vi "VariantSelection.vi"(8 "error in (no error)":errorcluster) -> (0 "error out":errorcluster, 2 "Cancelled":bool)   [LabVIEW 2013]
uses:
  <vilib>/addons/database/NI_Database_API.lvlib
  VariableLIB/Global.vi
  <vilib>/addons/database/Connection.llb/DB Tools Open Connec (String).vi
  Controls/AppleButton.ctl
panel:
  in  "Cancel":T1
  in  "Part":i32(ring) items=["HF DELUXE", "SPLENDOR PRO", "HF DELUXE WITH SIDE STAND", "SPLENDOR PRO WITH SIDE STAND", "CD DELUXE", "AAHC"]
  in  "OK":T1
  in  "Model":i32(ring) items=["AAHC", "DEFAULT MODEL", "HMCL"]
  # "Variant selection"
  # "Select a model"
  # "Select a part"
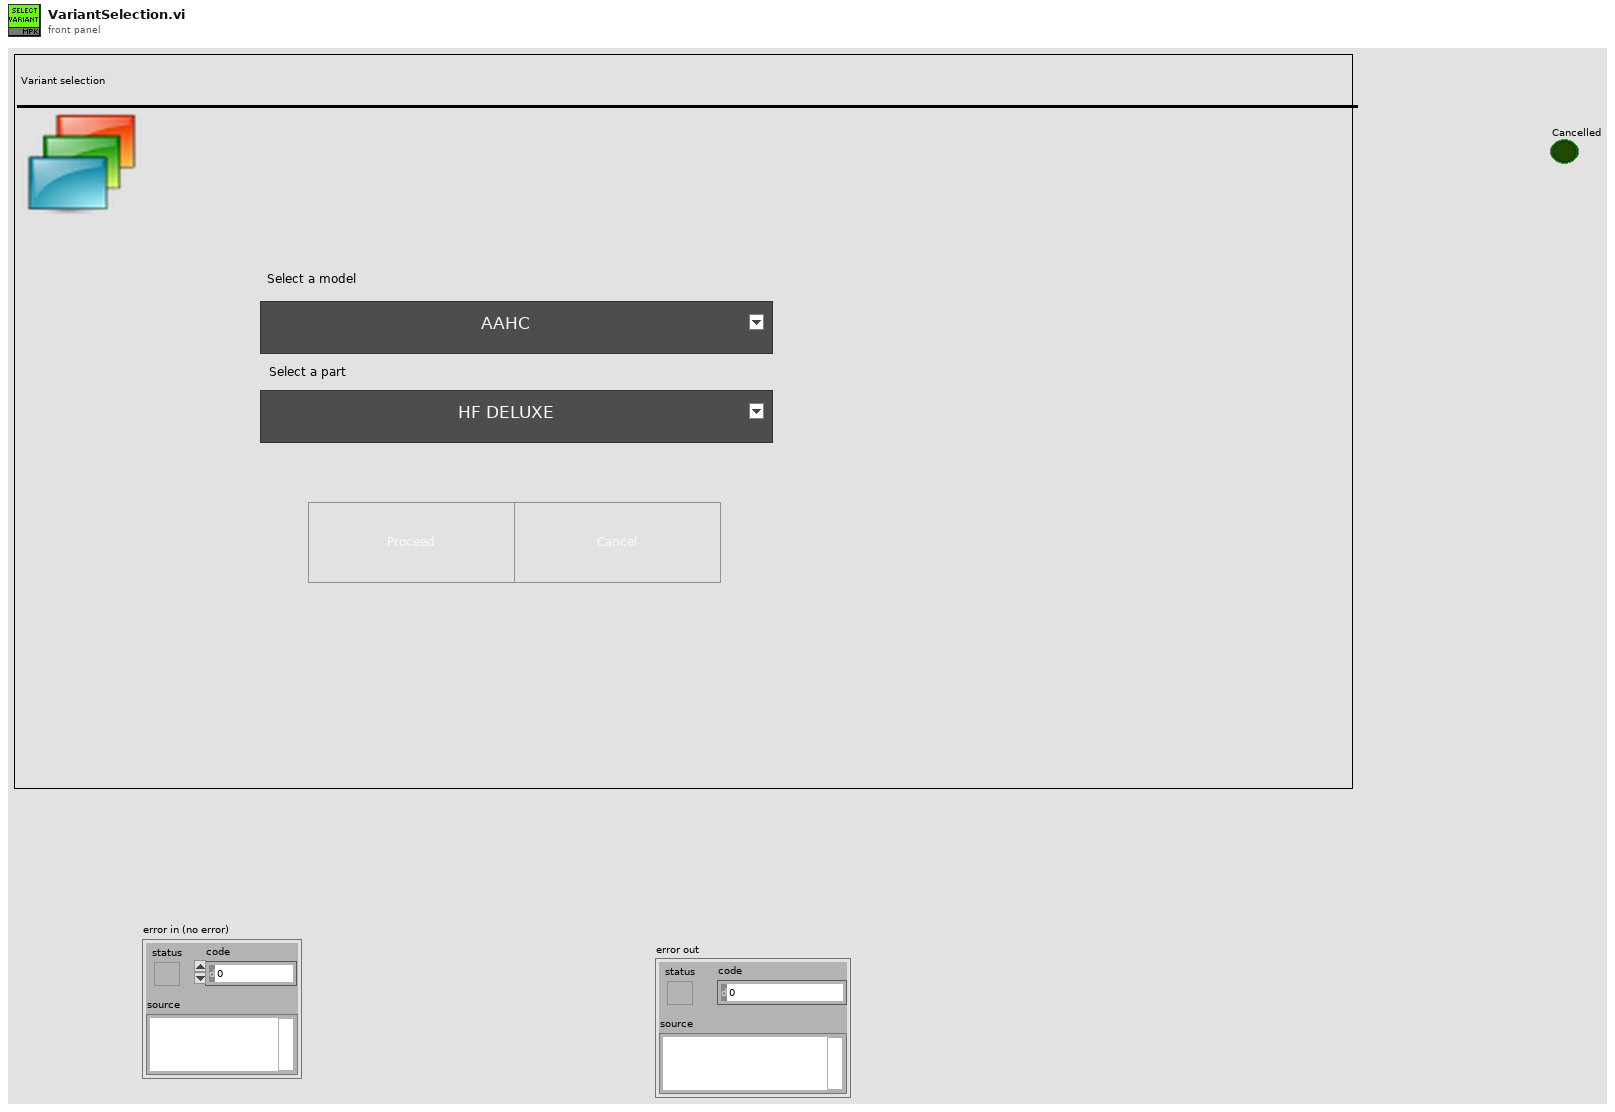
[diagram p1: front panel]
types:
  T1 = typedef "AppleButton.ctl" = bool
  T2 = typedef "NI_Database_API.lvlib/Conn ObjectReference.ctl" = refnum<k1>
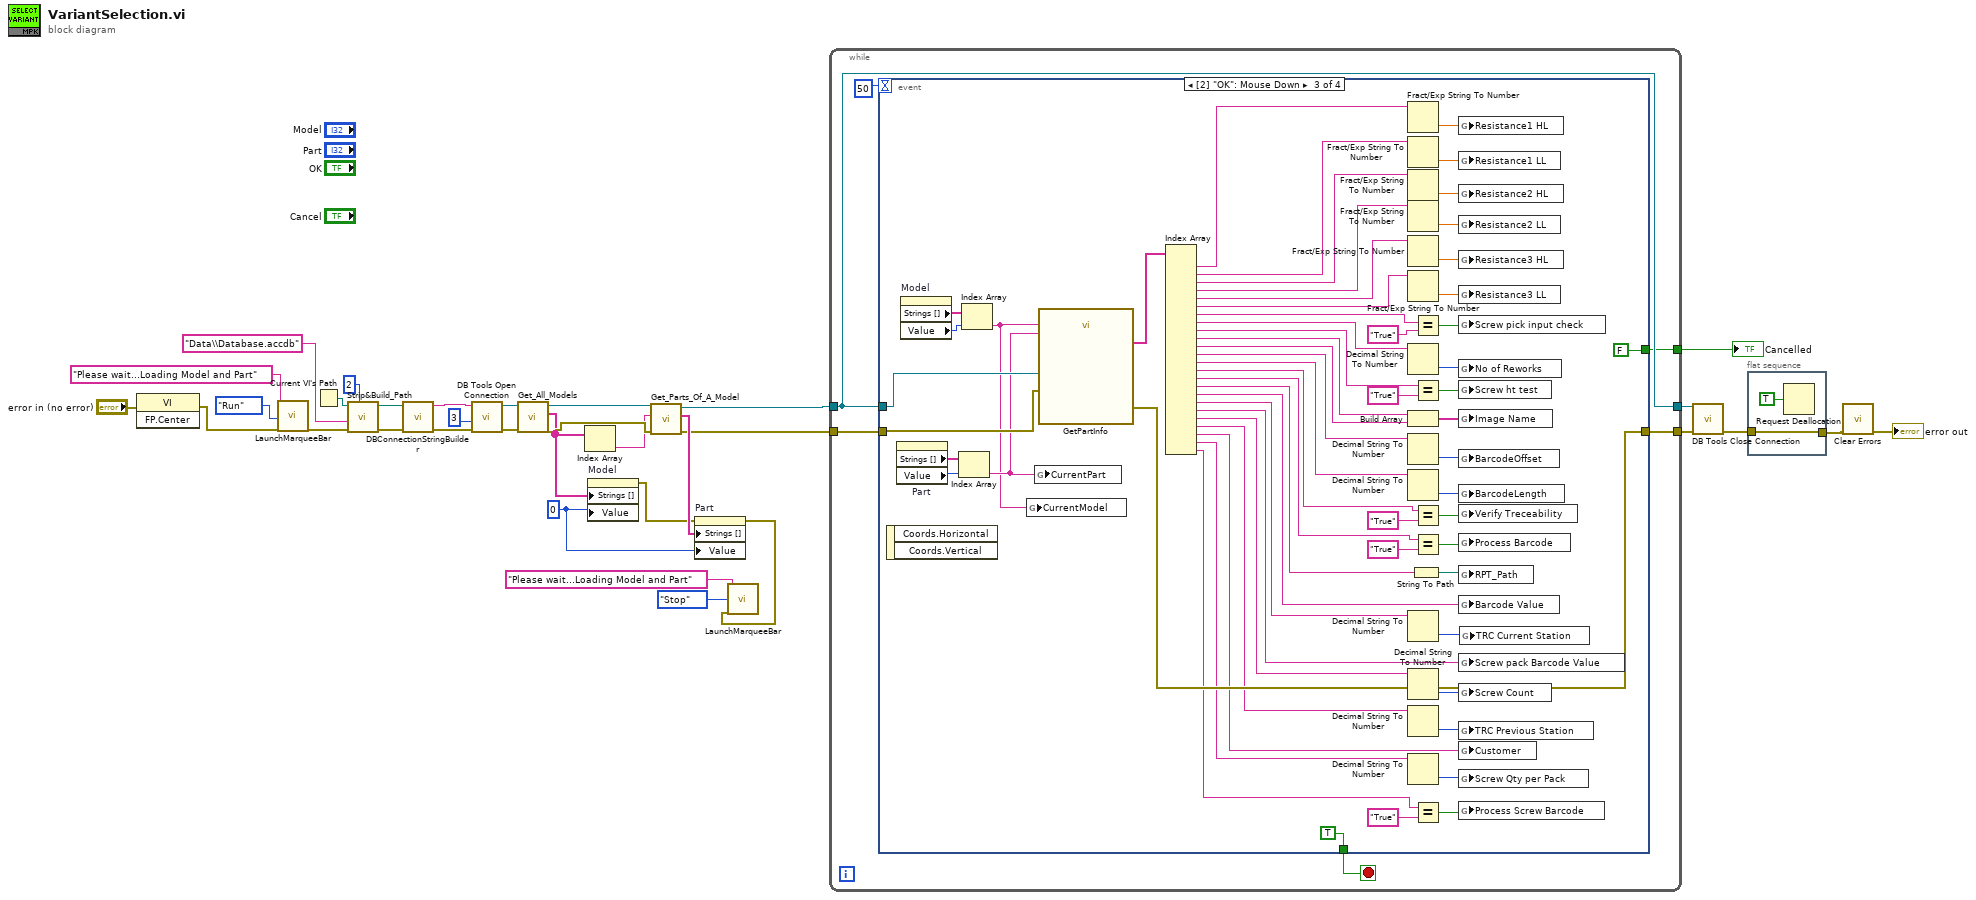
[diagram p0: block diagram]
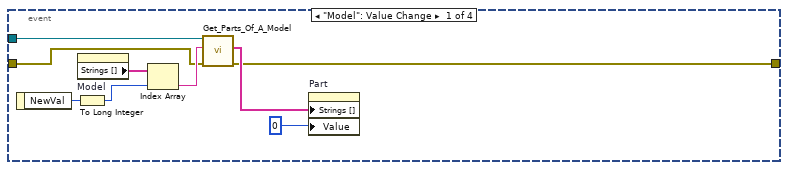
[diagram p2: hidden frame]
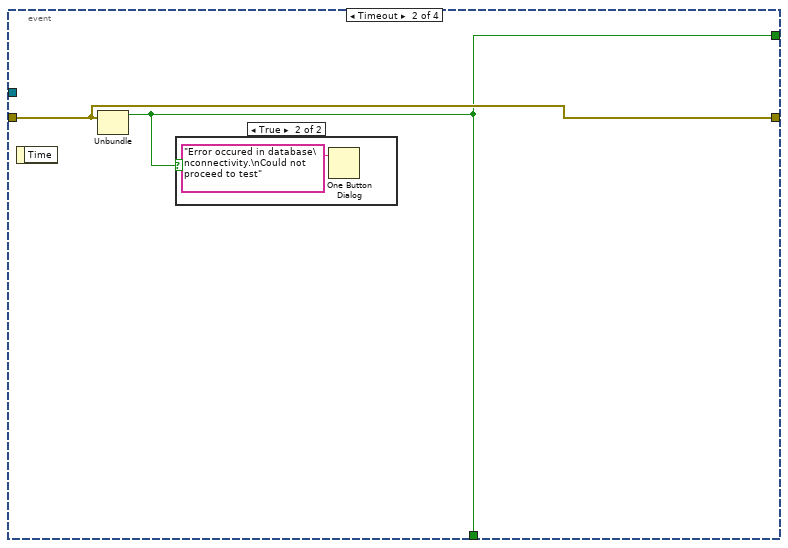
[diagram p3: hidden frame]
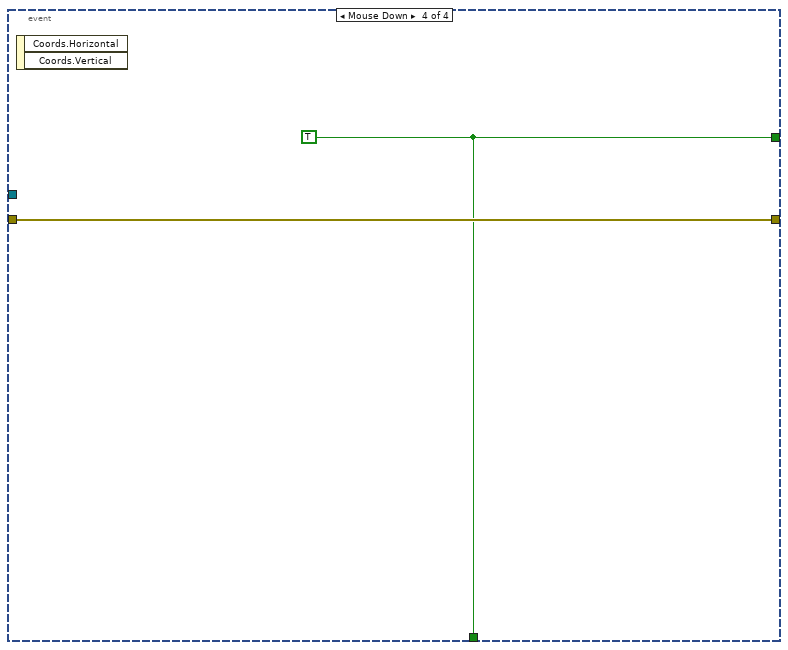
[diagram p5: hidden frame]
diagram:
  w18 = 0 ("connection timeout (15)")
  n1 = invoke class="VI" method="FP.Center"(error in="error in (no error)") -> (error out=w7:errorcluster)  [unwired: 2 in, 2 out]
  n2 = call "LaunchMarqueeBar.vi"("Action"=enum16{"Run", "EditMsg", "Stop"}."Run", "Message"="Please wait...Loading Model and Part", "error in (no error)"=w7) -> ("error out"=w4:errorcluster)  [unwired: 16 in]
  n3 = Current VI's Path() -> (path=w31:path)
  n4 = call "Strip&Build_Path.vi"("Strip_Levels"=2, "error in (no error)"=w4, "Build_Path"="Data\\Database.accdb", "Path_In"=w31) -> ("error out"=w12:errorcluster, "New_Path_Out"=w11:path)  [unwired: 5 in, 1 out]
  n5 = call "DBConnectionStringBuilder.vi"("error in"=w12, "DatabasePathIn"=w11) -> ("error out"=w9:errorcluster, "ConnectionStringOut"=w10:string)  [unwired: 8 in]
  n6 = call-poly <vilib>:"DB Tools Open Connection.vi"("error in (no error)"=w9, "connection timeout (15)"=3, "connection information"=w10) -> ("error out"=w28:errorcluster, "connection reference"=w29:T2)  [unwired: 5 in]
  n7 = call "Get_All_Models.vi"("error in (no error)"=w28, "DBRefnumIn"=w29) -> ("error out"=w26:errorcluster, "ModelsOut"=w24:string[], "DBRefnumOut"=w27:T2)  [unwired: 7 in]
  n8 = Index Array(array=w24) -> (element=w25:string)  [unwired: 1 in]
  n9 = property on="Model" class="Ring (strict)"("Strings []"=w24, "Value"=w18) -> (error out=w5:errorcluster)  [unwired: 2 in, 1 out]
  n10 = call "Get_Parts_Of_A_Model.vi"("error in (no error)"=w26, "Model"=w25, "DBRefnumIn"=w27) -> ("error out"=w21:errorcluster, "PartsOut"=w23:string[], "DBRefnumOut"=w22:T2)  [unwired: 6 in]
  n11 = property on="Part" class="Ring (strict)"(error in=w5, "Strings []"=w23, "Value"=w18) -> (error out=w1:errorcluster)  [unwired: 1 in, 1 out]
  n12 = call "LaunchMarqueeBar.vi"("Action"=enum16{"Run", "EditMsg", "Stop"}."Stop", "Message"="Please wait...Loading Model and Part", "error in (no error)"=w1) -> ()  [unwired: 16 in, 1 out]
  n13 = while {
    tunnel: w22 -> [w36]
    tunnel: w21 -> [w39]
    tunnel: [w38] -> w20
    tunnel: [w36] -> w19
    tunnel: [w35] -> w14
    stop <- w37 stop-if-true
    n14 = event shown="[2] \"OK\": Mouse Down" {
      selector: _ -> [_ _ _ _]
      dyn-events: _ -> [_ _ _ _]
      timeout: 50 -> [_ _ _ _]
      tunnel: w36 -> [w47 _ w112 _]
      tunnel: w39 -> [w42 w50 w111 w114]
      tunnel: [w41 w50 w103 w114] -> w38
      tunnel: [_ w49 TRUE w113] -> w37
      tunnel: [_ w49 FALSE ("status") w113] -> w35
      event "Model": Value Change {
        n15 = event-data() -> ("NewVal"=w45:i32)  [unwired: 1 in]
        n16 = To Long Integer(number=w45) -> (32bit integer=w43:i32)
        n17 = property on="Model" class="Ring (strict)"() -> ("Strings []"=w46:string[])  [unwired: 2 in, 2 out]
        n18 = Index Array(array=w46, index=w43) -> (element=w44:string)
        n19 = call "Get_Parts_Of_A_Model.vi"("error in (no error)"=w42, "Model"=w44, "DBRefnumIn"=w47) -> ("error out"=w41:errorcluster, "PartsOut"=w48:string[])  [unwired: 6 in, 1 out]
        n20 = property on="Part" class="Ring (strict)"("Strings []"=w48, "Value"=0 ("connection timeout (15)")) -> ()  [unwired: 2 in, 2 out]
      }
      event Timeout {
        n21 = event-data() -> ()  [unwired: 1 in, 1 out]
        n22 = Unbundle(w50) -> ("status"=w49:bool)  [unwired: 2 out]
        n23 = case shown="True" w49 {
          frame False {
          }
          frame True {
            n24 = One Button Dialog(message="Error occured in database\nconnectivity.\nCould not proceed to test") -> ()  [unwired: 1 in, 1 out]
          }
        }
      }
      event Mouse Down {
        n25 = event-data() -> ()  [unwired: 1 in, 2 out]
        n26 = property on="Part" class="Ring (strict)"() -> ("Strings []"=w108:string[], "Value"=w107:i32)  [unwired: 2 in, 2 out]
        n27 = property on="Model" class="Ring (strict)"() -> ("Strings []"=w109:string[], "Value"=w110:i32)  [unwired: 2 in, 2 out]
        n28 = Index Array(array=w108, index=w107) -> (element=w102:string)
        n29 = Index Array(array=w109, index=w110) -> (element=w97:string)
        n30 = global write "Global.vi" "CurrentModel"(w97) -> ()
        n31 = global write "Global.vi" "CurrentPart"(w102) -> ()
        n32 = call "GetPartInfo.vi"("error in (no error)"=w111, "Part"=w102, "Model"=w97, "DBRefnumIn"=w112) -> ("error out"=w103:errorcluster, "Data"=w98:string[])  [unwired: 4 in, 2 out]
        n33 = Index Array(array=w98) -> (element #1=w64:string, element #2=w63:string, element #3=w62:string, element #4=w61:string, element #5=w60:string, element #6=w59:string, element #7=w58:string, element #8=w57:string, element #9=w56:string, element #10=w54:string, element #11=w53:string, element #12=w91:string, element #13=w90:string, element #14=w75:string, element #15=w89:string, element #16=w88:string, element #17=w74:string, element #18=w72:string, element #19=w68:string, element #20=w87:string, element #21=w85:string, element #22=w71:string, element #23=w69:string, element #24=w65:string)  [unwired: 24 in]
        n34 = Fract/Exp String To Number(string=w64) -> (number=w78:dbl)  [unwired: 3 in, 1 out]
        n35 = Fract/Exp String To Number(string=w63) -> (number=w79:dbl)  [unwired: 3 in, 1 out]
        n36 = Fract/Exp String To Number(string=w62) -> (number=w80:dbl)  [unwired: 3 in, 1 out]
        n37 = Fract/Exp String To Number(string=w61) -> (number=w81:dbl)  [unwired: 3 in, 1 out]
        n38 = Fract/Exp String To Number(string=w60) -> (number=w82:dbl)  [unwired: 3 in, 1 out]
        n39 = Fract/Exp String To Number(string=w59) -> (number=w83:dbl)  [unwired: 3 in, 1 out]
        n40 = Decimal String To Number(string=w57) -> (number=w99:i32)  [unwired: 2 in, 1 out]
        n41 = Build Array(w54, w53) -> (w52:string[])
        n42 = Decimal String To Number(string=w91) -> (number=w106:i32)  [unwired: 2 in, 1 out]
        n43 = Decimal String To Number(string=w90) -> (number=w105:i32)  [unwired: 2 in, 1 out]
        n44 = Decimal String To Number(string=w72) -> (number=w73:i32)  [unwired: 2 in, 1 out]
        n45 = Decimal String To Number(string=w87) -> (number=w86:i32)  [unwired: 2 in, 1 out]
        n46 = Decimal String To Number(string=w85) -> (number=w84:i32)  [unwired: 2 in, 1 out]
        n47 = Decimal String To Number(string=w69) -> (number=w70:i32)  [unwired: 2 in, 1 out]
        n48 = String To Path(string=w88) -> (path=w104:path)
        n49 = Equal?(x=w58, y="True") -> (x = y?=w93:bool)
        n50 = Equal?(x=w56, y="True") -> (x = y?=w94:bool)
        n51 = Equal?(x=w75, y="True") -> (x = y?=w77:bool)
        n52 = Equal?(x=w89, y="True") -> (x = y?=w95:bool)
        n53 = Equal?(x=w65, y="True") -> (x = y?=w67:bool)
        n54 = global write "Global.vi" "Resistance1 HL"(w78) -> ()
        n55 = global write "Global.vi" "Resistance1 LL"(w79) -> ()
        n56 = global write "Global.vi" "Resistance2 HL"(w80) -> ()
        n57 = global write "Global.vi" "Resistance2 LL"(w81) -> ()
        n58 = global write "Global.vi" "Resistance3 HL"(w82) -> ()
        n59 = global write "Global.vi" "Resistance3 LL"(w83) -> ()
        n60 = global write "Global.vi" "Screw pick input check"(w93) -> ()
        n61 = global write "Global.vi" "No of Reworks"(w99) -> ()
        n62 = global write "Global.vi" "Screw ht test"(w94) -> ()
        n63 = global write "Global.vi" "Image Name"(w52) -> ()
        n64 = global write "Global.vi" "BarcodeOffset"(w106) -> ()
        n65 = global write "Global.vi" "BarcodeLength"(w105) -> ()
        n66 = global write "Global.vi" "Verify Treceability"(w77) -> ()
        n67 = global write "Global.vi" "Process Barcode"(w95) -> ()
        n68 = global write "Global.vi" "RPT_Path"(w104) -> ()
        n69 = global write "Global.vi" "Barcode Value"(w74) -> ()
        n70 = global write "Global.vi" "Screw pack Barcode Value"(w68) -> ()
        n71 = global write "Global.vi" "Screw Count"(w86) -> ()
        n72 = global write "Global.vi" "TRC Previous Station"(w84) -> ()
        n73 = global write "Global.vi" "Customer"(w71) -> ()
        n74 = global write "Global.vi" "Screw Qty per Pack"(w70) -> ()
        n75 = global write "Global.vi" "Process Screw Barcode"(w67) -> ()
        n76 = global write "Global.vi" "TRC Current Station"(w73) -> ()
      }
      event Mouse Down {
        w113 = TRUE ("status")
        n77 = event-data() -> ()  [unwired: 1 in, 2 out]
      }
    }
  }
  "Cancelled" <- w14
  n78 = call <vilib>:"DB Tools Close Connection.vi"("error in (no error)"=w20, "connection reference"=w19) -> ("error out"=w17:errorcluster)  [unwired: 5 in]
  n79 = flat-sequence {
    tunnel: w17 -> [w115]
    tunnel: [w115] -> w16
    frame #0 {
      n80 = Request Deallocation(TRUE ("flag")) -> ()
    }
  }
  n81 = call <vilib>:"Clear Errors.vi"("error in (no error)"=w16) -> ("error out"=→"error out":errorcluster)  [unwired: 5 in, 1 out]
